vi "ElevatorStateControl.vi"(9 "Elevator State":string) -> (1 "Elevator State Out":string, 2 "Target Elevator Position":dbl, 4 "Target Vacuum Pump Power":dbl)   [LabVIEW 2018]
uses:
  Inputs_DriverStation.vi
  SensorReadings.vi
  RobotStates.vi
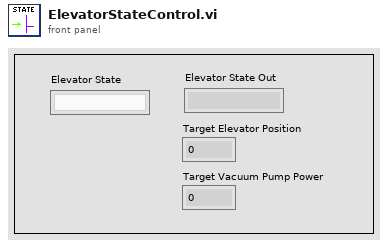
[diagram p1: front panel]
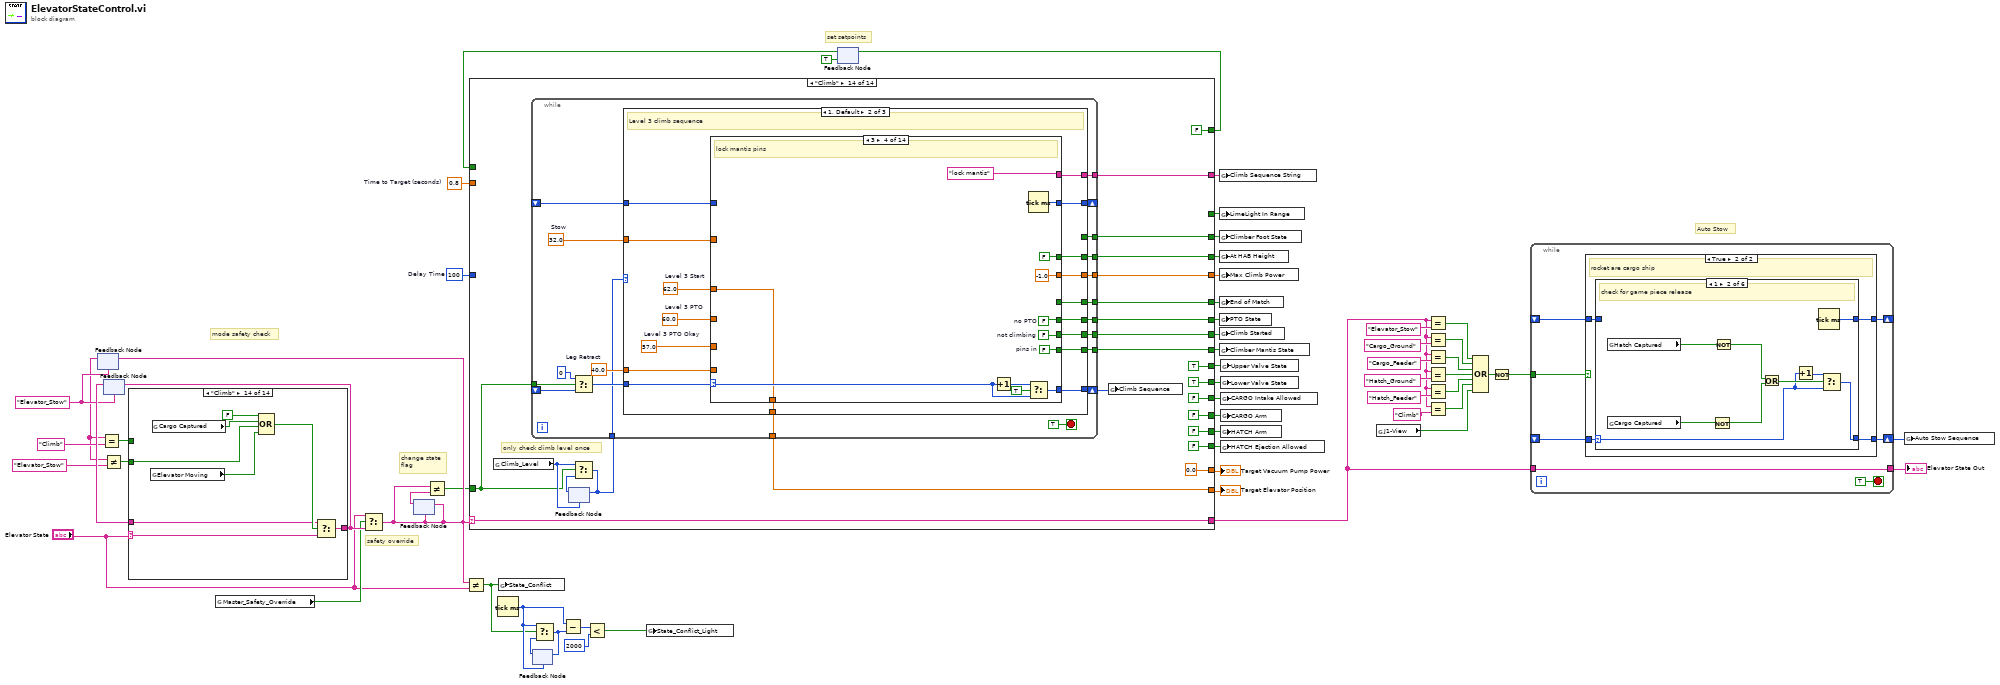
[diagram p0: block diagram]
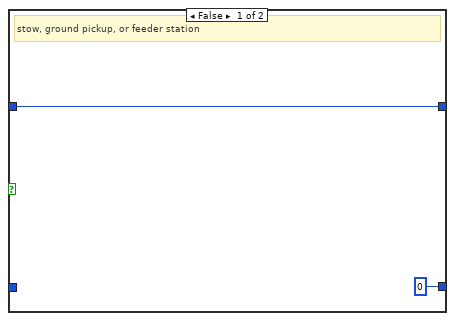
[diagram p2: hidden frame]
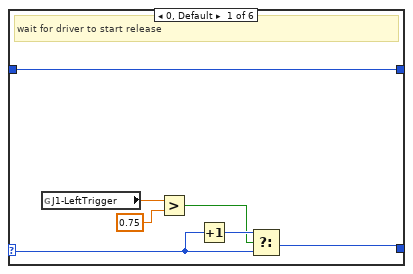
[diagram p3: hidden frame]
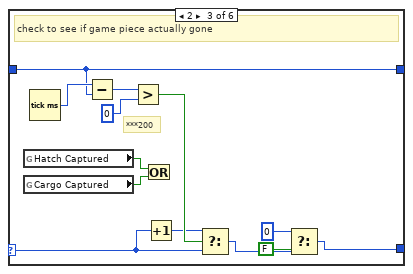
[diagram p4: hidden frame]
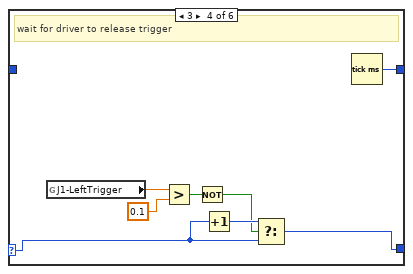
[diagram p5: hidden frame]
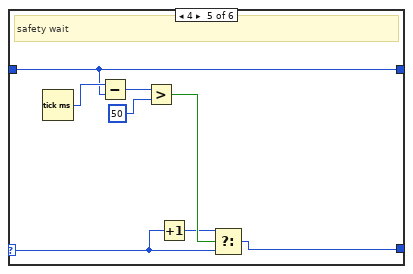
[diagram p6: hidden frame]
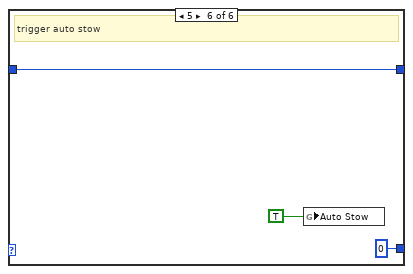
[diagram p7: hidden frame]
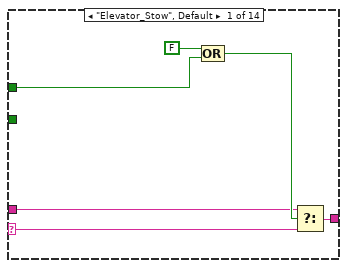
[diagram p8: hidden frame]
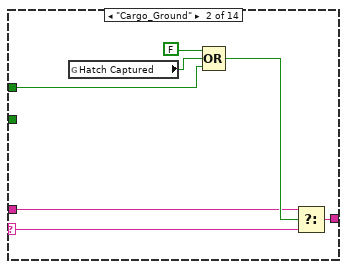
[diagram p9: hidden frame]
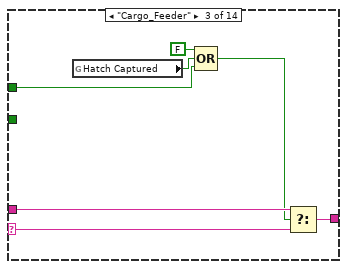
[diagram p10: hidden frame]
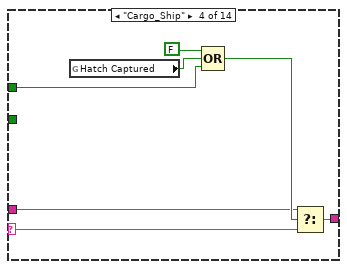
[diagram p11: hidden frame]
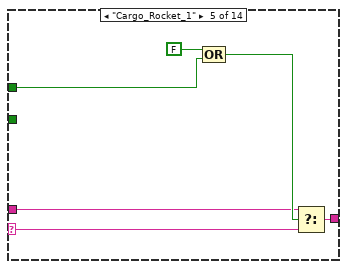
[diagram p12: hidden frame]
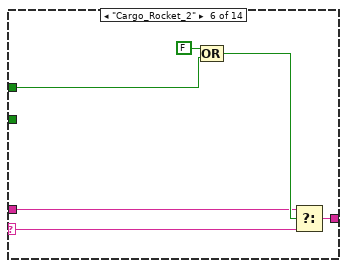
[diagram p13: hidden frame]
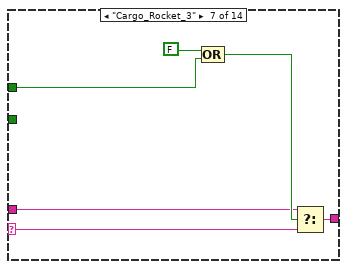
[diagram p14: hidden frame]
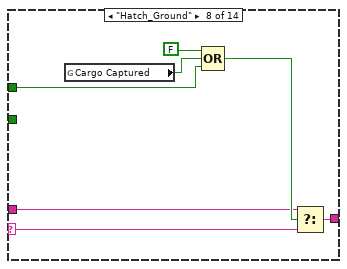
[diagram p15: hidden frame]
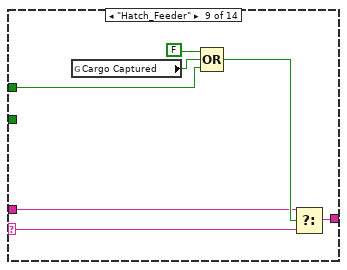
[diagram p16: hidden frame]
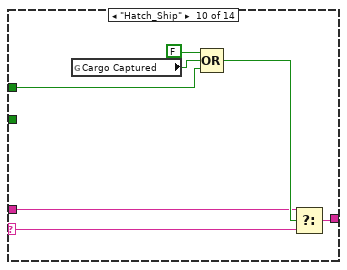
[diagram p17: hidden frame]
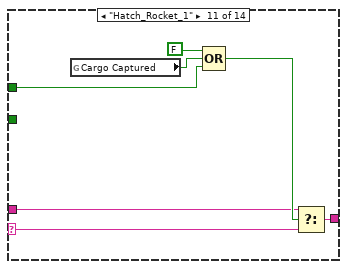
[diagram p18: hidden frame]
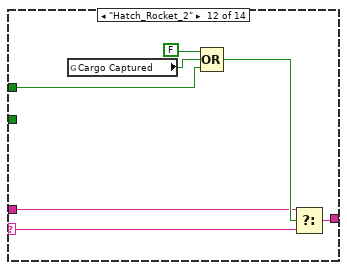
[diagram p19: hidden frame]
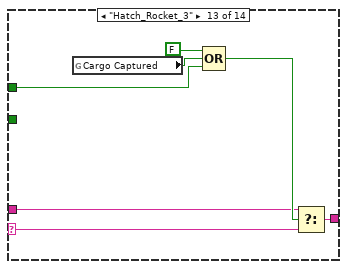
[diagram p20: hidden frame]
diagram:
  w3 = u32 100  # Delay Time
  w4 = 0.8  # Time to Target (seconds)
  w46 = "Elevator_Stow" ("Elevator State")
  # "change state\nflag"
  # "Auto Stow"
  # "safety override"
  # "mode safety check"
  # "set setpoints"
  n1 = feedback #1(w46) -> (w11:string)
  n2 = Equal?(x=w11, y="Climb") -> (x = y?=w47:bool)
  n3 = feedback #2(w46) -> (w49:string)
  n4 = Not Equal?(x=w11, y="Elevator_Stow") -> (x != y?=w10:bool)
  n5 = case shown="\"Climb\"" "Elevator State" {
    selector: "Elevator State" -> [w62 w69 w80 w83 w89 w95 w102 w108 w115 w122 w129 w136 w144 w151]
    tunnel: [w64 w71 w79 w85 w91 w97 w103 w110 w117 w124 w131 w138 w145 w152] -> w54
    tunnel: w49 -> [w63 w70 w78 w84 w90 w96 w101 w109 w116 w123 w130 w137 w143 w150]
    tunnel: w47 -> [w61 w67 w74 w81 w88 w94 w100 w106 w113 w120 w127 w134 w141 _]
    tunnel: w10 -> [_ _ _ _ _ _ _ _ _ _ _ _ _ w149]
    frame "Elevator_Stow", Default {
      n6 = Compound Arithmetic op=OR(FALSE, w61) -> (w65:bool)
      n7 = Select(t=w63, s=w65, f=w62) -> (s? t:f=w64:string)
    }
    frame "Cargo_Ground" {
      n8 = global read "SensorReadings.vi" "Hatch Captured"() -> (w68:bool)
      n9 = Compound Arithmetic op=OR(FALSE, w68, w67) -> (w72:bool)
      n10 = Select(t=w70, s=w72, f=w69) -> (s? t:f=w71:string)
    }
    frame "Cargo_Feeder" {
      n11 = global read "SensorReadings.vi" "Hatch Captured"() -> (w75:bool)
      n12 = Compound Arithmetic op=OR(FALSE, w75, w74) -> (w76:bool)
      n13 = Select(t=w78, s=w76, f=w80) -> (s? t:f=w79:string)
    }
    frame "Cargo_Ship" {
      n14 = global read "SensorReadings.vi" "Hatch Captured"() -> (w82:bool)
      n15 = Compound Arithmetic op=OR(FALSE, w82, w81) -> (w86:bool)
      n16 = Select(t=w84, s=w86, f=w83) -> (s? t:f=w85:string)
    }
    frame "Cargo_Rocket_1" {
      n17 = Compound Arithmetic op=OR(FALSE, w88) -> (w92:bool)
      n18 = Select(t=w90, s=w92, f=w89) -> (s? t:f=w91:string)
    }
    frame "Cargo_Rocket_2" {
      n19 = Compound Arithmetic op=OR(FALSE, w94) -> (w98:bool)
      n20 = Select(t=w96, s=w98, f=w95) -> (s? t:f=w97:string)
    }
    frame "Cargo_Rocket_3" {
      n21 = Compound Arithmetic op=OR(FALSE, w100) -> (w104:bool)
      n22 = Select(t=w101, s=w104, f=w102) -> (s? t:f=w103:string)
    }
    frame "Hatch_Ground" {
      n23 = global read "SensorReadings.vi" "Cargo Captured"() -> (w107:bool)
      n24 = Compound Arithmetic op=OR(FALSE, w107, w106) -> (w111:bool)
      n25 = Select(t=w109, s=w111, f=w108) -> (s? t:f=w110:string)
    }
    frame "Hatch_Feeder" {
      n26 = global read "SensorReadings.vi" "Cargo Captured"() -> (w114:bool)
      n27 = Compound Arithmetic op=OR(FALSE, w114, w113) -> (w118:bool)
      n28 = Select(t=w116, s=w118, f=w115) -> (s? t:f=w117:string)
    }
    frame "Hatch_Ship" {
      n29 = global read "SensorReadings.vi" "Cargo Captured"() -> (w121:bool)
      n30 = Compound Arithmetic op=OR(FALSE, w121, w120) -> (w125:bool)
      n31 = Select(t=w123, s=w125, f=w122) -> (s? t:f=w124:string)
    }
    frame "Hatch_Rocket_1" {
      n32 = global read "SensorReadings.vi" "Cargo Captured"() -> (w128:bool)
      n33 = Compound Arithmetic op=OR(FALSE, w128, w127) -> (w132:bool)
      n34 = Select(t=w130, s=w132, f=w129) -> (s? t:f=w131:string)
    }
    frame "Hatch_Rocket_2" {
      n35 = global read "SensorReadings.vi" "Cargo Captured"() -> (w135:bool)
      n36 = Compound Arithmetic op=OR(FALSE, w135, w134) -> (w139:bool)
      n37 = Select(t=w137, s=w139, f=w136) -> (s? t:f=w138:string)
    }
    frame "Hatch_Rocket_3" {
      n38 = global read "SensorReadings.vi" "Cargo Captured"() -> (w142:bool)
      n39 = Compound Arithmetic op=OR(FALSE, w142, w141) -> (w146:bool)
      n40 = Select(t=w143, s=w146, f=w144) -> (s? t:f=w145:string)
    }
    frame "Climb" {
      n41 = global read "RobotStates.vi" "Elevator Moving"() -> (w148:bool)
      n42 = global read "SensorReadings.vi" "Cargo Captured"() -> (w153:bool)
      n43 = Compound Arithmetic op=OR(FALSE, w153, w149, w148) -> (w154:bool)
      n44 = Select(t=w150, s=w154, f=w151) -> (s? t:f=w152:string)
    }
  }
  n45 = feedback-in #2(w54) -> ()
  n46 = global read "Inputs_DriverStation.vi" "Master_Safety_Override"() -> (w53:bool)
  n47 = Select(t="Elevator State", s=w53, f=w54) -> (s? t:f=w16:string)
  n48 = feedback-in #1(w16) -> ()
  n49 = feedback-in #3(w16) -> ()
  n50 = feedback #3(w16) -> (w17:string)
  n51 = Not Equal?(x=w16, y=w17) -> (x != y?=w15:bool)
  n52 = Not Equal?(x=w16, y="Elevator State") -> (x != y?=w22:bool)
  n53 = Tick Count (ms)() -> (millisecond timer value=w26:u32)
  n54 = global write "RobotStates.vi" "State_Conflict"(w22) -> ()
  n55 = feedback #4(w26) -> (w27:u32)
  n56 = Select(t=w26, s=w22, f=w27) -> (s? t:f=w25:u32)
  n57 = feedback-in #4(w25) -> ()
  n58 = Subtract(x=w26, y=w25) -> (x-y=w24:u32)
  n59 = Less?(x=w24, y=u32 2000) -> (x < y?=w21:bool)
  n60 = global write "RobotStates.vi" "State_Conflict_Light"(w21) -> ()
  n61 = feedback #5(TRUE) -> (w19:bool)
  n62 = case shown="\"Climb\"" w16 {
    selector: w16 -> [w179 w194 w234 w248 w289 w311 w333 w347 w409 w450 w491 w506 w521 w546]
    tunnel: [FALSE TRUE TRUE TRUE TRUE TRUE TRUE FALSE FALSE FALSE FALSE FALSE FALSE FALSE] -> w60
    tunnel: [w179 w194 w234 w248 w289 w311 w333 w347 w409 w450 w491 w506 w521 w546] -> w29
    tunnel: [w157 FALSE w197 TRUE TRUE w292 w315 FALSE FALSE FALSE FALSE FALSE FALSE FALSE] -> w59
    tunnel: [w178 32.0 w204 46.0 w275 w296 w313 32.0 w374 w436 w477 61.5 91.0 w532] -> w58
    tunnel: [FALSE FALSE FALSE FALSE FALSE FALSE FALSE TRUE w378 TRUE TRUE TRUE TRUE FALSE] -> w57
    tunnel: [w170 0.0 0.0 0.0 0.0 0.0 0.0 w343 w407 w448 w489 w502 w517 0.0 ("Vacuum_Pump")] -> w55
    tunnel: [FALSE FALSE FALSE FALSE FALSE FALSE FALSE TRUE TRUE TRUE TRUE TRUE TRUE FALSE] -> w56
    tunnel: [TRUE TRUE TRUE TRUE TRUE TRUE TRUE TRUE FALSE FALSE FALSE FALSE FALSE TRUE] -> w52
    tunnel: [TRUE TRUE TRUE TRUE TRUE TRUE TRUE FALSE TRUE TRUE TRUE TRUE TRUE TRUE] -> w51
    tunnel: [FALSE FALSE FALSE FALSE FALSE FALSE FALSE FALSE FALSE FALSE FALSE FALSE FALSE w535] -> w1
    tunnel: [w168 FALSE FALSE FALSE FALSE FALSE FALSE FALSE FALSE FALSE FALSE FALSE FALSE FALSE] -> w20
    tunnel: w19 -> [w164 _ _ _ _ _ _ _ _ _ _ _ _ _]
    tunnel: w15 -> [_ _ w212 _ _ _ _ _ w380 _ _ _ _ w534]
    tunnel: [w167 w184 w203 w238 w280 w303 w325 w338 w386 w443 w484 w497 w512 w531] -> w14
    tunnel: [w166 w183 w202 w237 w279 w302 w324 w337 w385 w442 w483 w496 w511 w530] -> w13
    tunnel: [FALSE FALSE FALSE FALSE FALSE FALSE FALSE FALSE FALSE FALSE FALSE FALSE FALSE w529] -> w9
    tunnel: [_ _ _ _ _ _ _ _ _ _ _ _ _ w527] -> w8
    tunnel: [-1.0 ("y") -1.0 ("y") -1.0 ("y") -1.0 ("y") -1.0 ("y") -1.0 ("y") -1.0 ("y") -1.0 ("y") -1.0 ("y") -1.0 ("y") -1.0 ("y") -1.0 ("y") -1.0 ("y") w526] -> w7
    tunnel: [_ _ _ _ _ _ _ _ _ _ _ _ _ w525] -> w6
    tunnel: [_ _ _ _ w267 _ _ _ w367 w429 w470 _ _ _] -> w5
    tunnel: w4 -> [_ _ _ _ w265 _ _ _ w365 w428 w468 _ _ _]
    tunnel: w3 -> [_ _ _ _ w266 _ _ _ w366 w427 w469 _ _ _]
    tunnel: [_ _ _ _ _ _ _ _ _ _ _ _ _ w524] -> w2
    frame "Elevator_Stow", Default {
      w166 = FALSE  # no PTO
      w167 = FALSE  # not climbing
      w178 = 32.0  # below 34.5 to ensure reset
      n63 = global read "Inputs_DriverStation.vi" "Reinit_Stow_Vacuum"() -> (w161:bool)
      n64 = global read "Inputs_DriverStation.vi" "Vacuum_Pump"() -> (w172:dbl)
      n65 = global read "RobotStates.vi" "Autopilot"() -> (w160:bool)
      n66 = Select(t=TRUE, s=w161, f=w164) -> (s? t:f=w163:bool)
      n67 = Select(t=w172, s=w163, f=0.0) -> (s? t:f=w170:dbl)
      n68 = Select(t=TRUE, s=w163, f=w163) -> (s? t:f=w168:bool)
      n69 = Select(t=TRUE, s=w160, f=FALSE) -> (s? t:f=w157:bool)
    }
    frame "Cargo_Ground" {
      w183 = FALSE  # no PTO
      w184 = FALSE  # not climbing
    }
    frame "Cargo_Feeder" {
      w199 = TRUE  # hold CARGO arm up
      w202 = FALSE  # no PTO
      w203 = FALSE  # not climbing
      w205 = 32.0  # gotten CARGO
      w209 = FALSE  # gotten CARGO
      w221 = -2.0  # (ft/s)
      w208 = 52.0  # getting CARGO
      w210 = TRUE  # getting CARGO
      # "autopilot"
      # "auto protect CARGO"
      n70 = global read "SensorReadings.vi" "EncoderVel_RightDrive"() -> (w225:dbl)
      n71 = global read "SensorReadings.vi" "EncoderVel_LeftDrive"() -> (w226:dbl)
      n72 = global read "SensorReadings.vi" "Cargo Captured"() -> (w219:bool)
      n73 = Add(x=w226, y=w225) -> (x+y=w224:dbl)
      n74 = Divide(x=w224, y=2.0) -> (x/y=w222:dbl)
      n75 = Less?(x=w222, y=w221) -> (x < y?=w220:bool)
      n76 = And(x=w220, y=w219) -> (x .and. y?=w218:bool)
      n77 = feedback #6(FALSE) -> (w216:bool)
      n78 = Select(t=TRUE, s=w218, f=w216) -> (s? t:f=w214:bool)
      n79 = Select(t=FALSE, s=w212, f=w214) -> (s? t:f=w207:bool)
      n80 = feedback-in #6(w207) -> ()
      n81 = Not(x=w207) -> (.not. x?=w206:bool)
      n82 = global read "RobotStates.vi" "Autopilot"() -> (w200:bool)
      n83 = Select(t=w210, s=w206, f=w209) -> (s? t:f=w198:bool)
      n84 = Select(t=w199, s=w200, f=w198) -> (s? t:f=w197:bool)
      n85 = Select(t=w208, s=w206, f=w205) -> (s? t:f=w204:dbl)
    }
    frame "Cargo_Ship" {
      w237 = FALSE  # no PTO
      w238 = FALSE  # not climbing
    }
    frame "Cargo_Rocket_1" {
      w256 = 1.5  # feet per second
      w279 = FALSE  # no PTO
      w280 = FALSE  # not climbing
      n86 = global read "SensorReadings.vi" "LimeLight Distance (in)"() -> (w254:dbl)
      n87 = global read "SensorReadings.vi" "EncoderVel_RightDrive"() -> (w263:dbl)
      n88 = global read "SensorReadings.vi" "EncoderVel_LeftDrive"() -> (w264:dbl)
      n89 = Add(x=w264, y=w263) -> (x+y=w262:dbl)
      n90 = Divide(x=w254, y=12.0) -> (x/y=w252:dbl)
      n91 = Divide(x=w262, y=2.0) -> (x/y=w257:dbl)
      n92 = In Range and Coerce(upper limit=10.0, x=w257, lower limit=w256) -> (coerced(x)=w255:dbl)  [unwired: 1 out]
      n93 = Divide(x=w252, y=w255) -> (x/y=w259:dbl)
      n94 = Greater Than 0?(x=w259) -> (x > 0?=w260:bool)
      n95 = Select(t=w259, s=w260, f=inf) -> (s? t:f=w251:dbl)
      n96 = global read "SensorReadings.vi" "LimeLight Valid"() -> (w270:bool)
      n97 = Select(t=w251, s=w270, f=inf) -> (s? t:f=w269:dbl)
      n98 = call "TimeBelowThreshold.vi"("Current Value"=w269, "Threshold"=w265) -> ("Time Below"=w271:u32)  [unwired: 3 in]
      n99 = global read "RobotStates.vi" "Autopilot"() -> (w277:bool)
      n100 = Greater?(x=w271, y=w266) -> (0:w272:bool)
      n101 = call "RisingEdgeTrigger.vi"("Raw Signal"=w272) -> ("Trigger"=w267:bool)
      n102 = Select(t=45.0, s=w277, f=32.0) -> (s? t:f=w275:dbl)
    }
    frame "Cargo_Rocket_2" {
      w302 = FALSE  # no PTO
      w303 = FALSE  # not climbing
      w296 = 62.5
      n103 = global read "SensorReadings.vi" "EncoderPos_Elevator"() -> (w297:dbl)
      n104 = Subtract(x=w297, y=w296) -> (x-y=w295:dbl)
      n105 = Absolute Value(x=w295) -> (abs(x)=w291:dbl)
      n106 = Less?(x=w291, y=10.0) -> (x < y?=w293:bool)
      n107 = Select(t=TRUE, s=w293, f=FALSE) -> (s? t:f=w292:bool)
    }
    frame "Cargo_Rocket_3" {
      w324 = FALSE  # no PTO
      w325 = FALSE  # not climbing
      w313 = 91.0
      n108 = global read "SensorReadings.vi" "EncoderPos_Elevator"() -> (w319:dbl)
      n109 = Subtract(x=w319, y=w313) -> (x-y=w318:dbl)
      n110 = Absolute Value(x=w318) -> (abs(x)=w316:dbl)
      n111 = Less?(x=w316, y=10.0) -> (x < y?=w317:bool)
      n112 = Select(t=TRUE, s=w317, f=FALSE) -> (s? t:f=w315:bool)
    }
    frame "Hatch_Ground" {
      w337 = FALSE  # no PTO
      w338 = FALSE  # not climbing
      n113 = global read "Inputs_DriverStation.vi" "Vacuum_Pump"() -> (w343:dbl)
    }
    frame "Hatch_Feeder" {
      w355 = 2.0  # feet per second
      w385 = FALSE  # no PTO
      w386 = FALSE  # not climbing
      w396 = -2.0  # (ft/s)
      w388 = FALSE  # gotten HATCH
      w402 = TRUE  # to get HATCH
      # "auto protect HATCH"
      n114 = global read "SensorReadings.vi" "EncoderVel_RightDrive"() -> (w400:dbl)
      n115 = global read "SensorReadings.vi" "EncoderVel_LeftDrive"() -> (w401:dbl)
      n116 = global read "SensorReadings.vi" "LimeLight Distance (in)"() -> (w353:dbl)
      n117 = global read "SensorReadings.vi" "EncoderVel_RightDrive"() -> (w363:dbl)
      n118 = global read "SensorReadings.vi" "EncoderVel_LeftDrive"() -> (w364:dbl)
      n119 = global read "SensorReadings.vi" "Hatch Captured"() -> (w382:bool)
      n120 = Add(x=w401, y=w400) -> (x+y=w399:dbl)
      n121 = Divide(x=w399, y=2.0) -> (x/y=w397:dbl)
      n122 = Less?(x=w397, y=w396) -> (x < y?=w395:bool)
      n123 = Add(x=w364, y=w363) -> (x+y=w362:dbl)
      n124 = And(x=w395, y=w382) -> (x .and. y?=w394:bool)
      n125 = Not(x=w382) -> (.not. x?=w381:bool)
      n126 = Divide(x=w353, y=12.0) -> (x/y=w351:dbl)
      n127 = Divide(x=w362, y=2.0) -> (x/y=w356:dbl)
      n128 = Or(x=w381, y=w380) -> (x .or. y?=w379:bool)
      n129 = feedback #7(FALSE) -> (w392:bool)
      n130 = Select(t=TRUE, s=w394, f=w392) -> (s? t:f=w390:bool)
      n131 = In Range and Coerce(upper limit=10.0 ("feet per second"), x=w356, lower limit=w355) -> (coerced(x)=w354:dbl)  [unwired: 1 out]
      n132 = Select(t=FALSE, s=w379, f=w390) -> (s? t:f=w387:bool)
      n133 = feedback-in #7(w387) -> ()
      n134 = Divide(x=w351, y=w354) -> (x/y=w359:dbl)
      n135 = Not(x=w387) -> (.not. x?=w383:bool)
      n136 = Greater Than 0?(x=w359) -> (x > 0?=w360:bool)
      n137 = Select(t=w359, s=w360, f=inf) -> (s? t:f=w357:dbl)
      n138 = global read "SensorReadings.vi" "LimeLight Valid"() -> (w371:bool)
      n139 = Select(t=w402, s=w383, f=w388) -> (s? t:f=w378:bool)
      n140 = Select(t=w357, s=w371, f=inf) -> (s? t:f=w372:dbl)
      n141 = global read "RobotStates.vi" "Autopilot"() -> (w377:bool)
      n142 = call "TimeBelowThreshold.vi"("Current Value"=w372, "Threshold"=w365) -> ("Time Below"=w369:u32)  [unwired: 3 in]
      n143 = global read "Inputs_DriverStation.vi" "Vacuum_Pump"() -> (w407:dbl)
      n144 = Greater?(x=w369, y=w366) -> (0:w368:bool)
      n145 = Select(t=55.0, s=w377, f=32.0) -> (s? t:f=w374:dbl)
      n146 = call "RisingEdgeTrigger.vi"("Raw Signal"=w368) -> ("Trigger"=w367:bool)
    }
    frame "Hatch_Ship" {
      w418 = 2.0  # feet per second
      w442 = FALSE  # no PTO
      w443 = FALSE  # not climbing
      n147 = global read "SensorReadings.vi" "LimeLight Distance (in)"() -> (w416:dbl)
      n148 = global read "SensorReadings.vi" "EncoderVel_RightDrive"() -> (w425:dbl)
      n149 = global read "SensorReadings.vi" "EncoderVel_LeftDrive"() -> (w426:dbl)
      n150 = Add(x=w426, y=w425) -> (x+y=w424:dbl)
      n151 = Divide(x=w416, y=12.0) -> (x/y=w414:dbl)
      n152 = Divide(x=w424, y=2.0) -> (x/y=w419:dbl)
      n153 = In Range and Coerce(upper limit=10.0, x=w419, lower limit=w418) -> (coerced(x)=w417:dbl)  [unwired: 1 out]
      n154 = Divide(x=w414, y=w417) -> (x/y=w421:dbl)
      n155 = Greater Than 0?(x=w421) -> (x > 0?=w422:bool)
      n156 = Select(t=w421, s=w422, f=inf) -> (s? t:f=w413:dbl)
      n157 = global read "SensorReadings.vi" "LimeLight Valid"() -> (w433:bool)
      n158 = Select(t=w413, s=w433, f=inf) -> (s? t:f=w434:dbl)
      n159 = call "TimeBelowThreshold.vi"("Current Value"=w434, "Threshold"=w428) -> ("Time Below"=w431:u32)  [unwired: 3 in]
      n160 = global read "RobotStates.vi" "Autopilot"() -> (w439:bool)
      n161 = global read "Inputs_DriverStation.vi" "Vacuum_Pump"() -> (w448:dbl)
      n162 = Greater?(x=w431, y=w427) -> (0:w430:bool)
      n163 = call "RisingEdgeTrigger.vi"("Raw Signal"=w430) -> ("Trigger"=w429:bool)
      n164 = Select(t=55.0, s=w439, f=32.0) -> (s? t:f=w436:dbl)
    }
    frame "Hatch_Rocket_1" {
      w459 = 2.0  # feet per second
      w483 = FALSE  # no PTO
      w484 = FALSE  # not climbing
      # "autopilot"
      n165 = global read "SensorReadings.vi" "LimeLight Distance (in)"() -> (w457:dbl)
      n166 = global read "SensorReadings.vi" "EncoderVel_RightDrive"() -> (w466:dbl)
      n167 = global read "SensorReadings.vi" "EncoderVel_LeftDrive"() -> (w467:dbl)
      n168 = Add(x=w467, y=w466) -> (x+y=w465:dbl)
      n169 = Divide(x=w457, y=12.0) -> (x/y=w455:dbl)
      n170 = Divide(x=w465, y=2.0) -> (x/y=w460:dbl)
      n171 = In Range and Coerce(upper limit=10.0, x=w460, lower limit=w459) -> (coerced(x)=w458:dbl)  [unwired: 1 out]
      n172 = Divide(x=w455, y=w458) -> (x/y=w462:dbl)
      n173 = Greater Than 0?(x=w462) -> (x > 0?=w463:bool)
      n174 = Select(t=w462, s=w463, f=inf) -> (s? t:f=w454:dbl)
      n175 = global read "SensorReadings.vi" "LimeLight Valid"() -> (w473:bool)
      n176 = Select(t=w454, s=w473, f=inf) -> (s? t:f=w472:dbl)
      n177 = call "TimeBelowThreshold.vi"("Current Value"=w472, "Threshold"=w468) -> ("Time Below"=w474:u32)  [unwired: 3 in]
      n178 = Greater?(x=w474, y=w469) -> (0:w475:bool)
      n179 = global read "RobotStates.vi" "Autopilot"() -> (w480:bool)
      n180 = global read "Inputs_DriverStation.vi" "Vacuum_Pump"() -> (w489:dbl)
      n181 = call "RisingEdgeTrigger.vi"("Raw Signal"=w475) -> ("Trigger"=w470:bool)
      n182 = Select(t=55.0, s=w480, f=32.0) -> (s? t:f=w477:dbl)
    }
    frame "Hatch_Rocket_2" {
      w496 = FALSE  # no PTO
      w497 = FALSE  # not climbing
      n183 = global read "Inputs_DriverStation.vi" "Vacuum_Pump"() -> (w502:dbl)
    }
    frame "Hatch_Rocket_3" {
      w511 = FALSE  # no PTO
      w512 = FALSE  # not climbing
      n184 = global read "Inputs_DriverStation.vi" "Vacuum_Pump"() -> (w517:dbl)
    }
    frame "Climb" {
      # "only check climb level once"
      n185 = global read "Inputs_DriverStation.vi" "Climb_Level"() -> (w536:u8)
      n186 = feedback #8(w536) -> (w537:u8)
      n187 = Select(t=w536, s=w534, f=w537) -> (s? t:f=w533:u8)
      n188 = while {
        shift-right: [w565] -> w528
        shift-left: _ -> [w561]
        shift-right: [w564] -> _
        shift-left: _ -> [w563]
        tunnel: [w562] -> w535
        tunnel: w534 -> [w559]
        tunnel: w533 -> [w552]
        tunnel: [w554] -> w532
        tunnel: [w557] -> w531
        tunnel: [w556] -> w530
        tunnel: [w555] -> w529
        tunnel: [w551] -> w527
        tunnel: [w550] -> w526
        tunnel: [w549] -> w525
        tunnel: [w547] -> w524
        stop <- TRUE stop-if-true
        w548 = 32.0  # Stow
        w553 = 40.0  # Leg Retract
        n189 = Select(t=0, s=w559, f=w561) -> (s? t:f=w560:i32)
        n190 = case shown="1, Default" w552 {
          tunnel: [w578 w831 w1054] -> w565
          tunnel: [w582 w838 w1061] -> w564
          tunnel: w563 -> [w584 w839 w1062]
          tunnel: [w577 w832 w1055] -> w562
          tunnel: w560 -> [w580 w837 w1060]
          tunnel: [w575 w833 w1056] -> w557
          tunnel: [w576 w834 w1057] -> w556
          tunnel: [w579 w835 w1058] -> w555
          tunnel: [w574 w830 w1053] -> w554
          tunnel: w553 -> [w581 w836 w1059]
          tunnel: [w583 w829 w1052] -> w551
          tunnel: [w573 w827 w1050] -> w550
          tunnel: [w572 w825 w1048] -> w549
          tunnel: w548 -> [w567 w824 w1047]
          tunnel: [_ _ w1046] -> w547
          frame 0 {
            w571 = 45.0  # Level 2 Pre-Climb
            w568 = 39.5  # Level 2 PTO Okay
            w570 = 45.5  # Level 2 Start
            w569 = 42.5  # Level 2 PTO
            # "Level 2 climb sequence"
            n191 = case shown="1" w580 {
              selector: w580 -> [w594 w609 w624 w641 w652 w673 w684 w703 w722 w733 w751 w760 w775 w787 w804 w818]
              tunnel: [w596 w611 w619 w640 w651 w672 w686 w705 w721 w732 w750 w759 w774 w786 w803 w818] -> w578
              tunnel: [w593 w599 w617 w638 w654 w665 w685 w704 w717 w725 w738 w763 w777 w789 w811 w821] -> w582
              tunnel: w584 -> [_ w599 w617 _ w654 w665 w685 w704 w717 _ w738 w763 w777 w789 w811 w821]
              tunnel: [w592 w608 w630 w639 w650 w675 w689 w708 w724 w735 w753 w764 w778 w790 w812 w822] -> w577
              tunnel: [w585 w597 w612 w631 w643 w658 _ w693 _ _ _ _ w770 w785 w806 w815] -> w574
              tunnel: [w590 w607 w618 w636 w649 w668 w690 w709 w720 w731 w749 w765 w779 w791 w813 w823] -> w575
              tunnel: [w589 w606 w616 w635 w648 w667 w691 w710 w719 w730 w748 w758 w773 w783 w809 w819] -> w576
              tunnel: [FALSE FALSE FALSE FALSE FALSE FALSE FALSE FALSE FALSE FALSE FALSE w762 TRUE TRUE TRUE FALSE] -> w579
              tunnel: w581 -> [_ _ _ _ _ _ _ _ _ _ _ _ w770 w785 w806 w815]
              tunnel: ["release mantis" "wait for mantis to deploy" "wait for elevator to reach climb height" "lock mantis" "confirm mantis lock" "wait for the driver to start climbing #1" "wait for driver to raise elevator" "wait for elevator to reach start height" "wait for elevator to pass PTO height" "engage the PTO" "ensure PTO is engaged" "wait for the robot to be on HAB" "stop climbing" "wait to disengage PTO" "retract the legs after confirm " "elevator powered down"] -> w583
              tunnel: [-1.0 ("y") -1.0 ("y") -1.0 ("y") -1.0 ("y") -1.0 ("y") -1.0 ("y") -1.0 ("y") -1.0 ("y") -0.05 ("y") -0.05 ("y") -0.05 ("y") -1.0 ("y") -1.0 ("y") -1.0 ("y") -1.0 ("y") -1.0 ("y")] -> w573
              tunnel: [_ _ _ _ _ _ _ _ _ _ _ _ _ _ _ w814] -> w572
              tunnel: w571 -> [_ _ w612 w631 w643 w658 _ _ _ _ _ _ _ _ _ _]
              tunnel: w570 -> [_ _ _ _ _ _ _ w693 _ _ _ _ _ _ _ _]
              tunnel: w569 -> [_ _ _ _ _ _ _ _ w712 _ _ _ _ _ _ _]
              tunnel: w568 -> [_ _ _ _ _ _ _ _ _ _ w736 _ _ _ _ _]
              tunnel: w567 -> [w585 w597 _ _ _ _ _ _ _ _ _ _ _ _ _ _]
              frame 0, Default {
                w589 = FALSE  # no PTO
                w590 = FALSE  # not climbing
                w592 = TRUE  # pins out
                # "release mantis pins and command to climb height"
                n192 = Increment(x=w594) -> (x+1=w595:i32)
                n193 = Select(t=w595, s=TRUE, f=w594) -> (s? t:f=w596:i32)
                n194 = Tick Count (ms)() -> (millisecond timer value=w593:u32)
              }
              frame 1 {
                w606 = FALSE  # no PTO
                w607 = FALSE  # not climbing
                w608 = TRUE  # pins out
                # "wait for mantis to deploy"
                n195 = Tick Count (ms)() -> (millisecond timer value=w602:u32)
                n196 = Subtract(x=w602, y=w599) -> (x-y=w601:u32)
                n197 = Greater?(x=w601, y=u32 0) -> (0:w598:bool)
                n198 = Increment(x=w609) -> (x+1=w610:i32)
                n199 = Select(t=w610, s=w598, f=w609) -> (s? t:f=w611:i32)
              }
              frame 2 {
                w616 = FALSE  # no PTO
                w618 = FALSE  # not climbing
                w630 = TRUE  # pins out
                # "wait for elevator to start moving\nand then stop moving"
                # "wait for elevator to reach climb position"
                n200 = global read "RobotStates.vi" "Elevator Moving"() -> (w622:bool)
                n201 = call "RisingEdgeTrigger.vi"("Raw Signal"=w622) -> ("Trigger"=w629:bool)
                n202 = Not(x=w622) -> (.not. x?=w621:bool)
                n203 = feedback #9(FALSE) -> (w627:bool)
                n204 = Select(t=TRUE, s=w629, f=w627) -> (s? t:f=w623:bool)
                n205 = feedback-in #9(w623) -> ()
                n206 = And(x=w623, y=w621) -> (x .and. y?=w620:bool)
                n207 = Increment(x=w624) -> (x+1=w625:i32)
                n208 = Select(t=w625, s=w620, f=w624) -> (s? t:f=w619:i32)
              }
              frame 3 {
                w635 = FALSE  # no PTO
                w636 = FALSE  # not climbing
                w639 = FALSE  # pins in
                # "lock mantis pins"
                n209 = Increment(x=w641) -> (x+1=w642:i32)
                n210 = Tick Count (ms)() -> (millisecond timer value=w638:u32)
                n211 = Select(t=w642, s=TRUE, f=w641) -> (s? t:f=w640:i32)
              }
              frame 4 {
                w648 = FALSE  # no PTO
                w649 = FALSE  # not climbing
                w650 = FALSE  # pins in
                # "wait for mantis legs to lock"
                n212 = Tick Count (ms)() -> (millisecond timer value=w657:u32)
                n213 = Subtract(x=w657, y=w654) -> (x-y=w656:u32)
                n214 = Greater?(x=w656, y=u32 500) -> (0:w646:bool)
                n215 = Increment(x=w652) -> (x+1=w653:i32)
                n216 = Select(t=w653, s=w646, f=w652) -> (s? t:f=w651:i32)
              }
              frame 5 {
                w667 = FALSE  # no PTO
                w668 = FALSE  # not climbing
                w675 = FALSE  # pins in
                # "wait for the driver to start climbing"
                n217 = global read "Inputs_DriverStation.vi" "J1-RightTrigger"() -> (w664:dbl)
                n218 = Greater?(x=w664, y=0.2) -> (0:w662:bool)
                n219 = feedback #10(FALSE) -> (w669:bool)
                n220 = Select(t=TRUE, s=w662, f=w669) -> (s? t:f=w661:bool)
                n221 = feedback-in #10(w661) -> ()
                n222 = Increment(x=w673) -> (x+1=w674:i32)
                n223 = Select(t=w674, s=w661, f=w673) -> (s? t:f=w672:i32)
              }
              frame 6 {
                w691 = FALSE  # no PTO
                w690 = TRUE  # climbing
                w689 = FALSE  # pins in
                # "Lower elevator contacts HAB first time"
                n224 = global read "Inputs_DriverStation.vi" "J1-LeftTrigger"() -> (w680:dbl)
                n225 = Greater?(x=w680, y=0.75) -> (0:w678:bool)
                n226 = feedback #11(FALSE) -> (w681:bool)
                n227 = Select(t=TRUE, s=w678, f=w681) -> (s? t:f=w677:bool)
                n228 = feedback-in #11(w677) -> ()
                n229 = Increment(x=w684) -> (x+1=w687:i32)
                n230 = Select(t=w687, s=w677, f=w684) -> (s? t:f=w686:i32)
              }
              frame 7 {
                w710 = FALSE  # no PTO
                w709 = FALSE  # not climbing
                w708 = FALSE  # pins in
                # "Wait for elevator to reach start height"
                n231 = global read "RobotStates.vi" "Elevator Moving"() -> (w696:bool)
                n232 = call "RisingEdgeTrigger.vi"("Raw Signal"=w696) -> ("Trigger"=w701:bool)
                n233 = Not(x=w696) -> (.not. x?=w695:bool)
                n234 = feedback #12(FALSE) -> (w699:bool)
                n235 = Select(t=TRUE, s=w701, f=w699) -> (s? t:f=w697:bool)
                n236 = feedback-in #12(w697) -> ()
                n237 = And(x=w697, y=w695) -> (x .and. y?=w694:bool)
                n238 = Increment(x=w703) -> (x+1=w706:i32)
                n239 = Select(t=w706, s=w694, f=w703) -> (s? t:f=w705:i32)
              }
              frame 8 {
                w719 = FALSE  # no PTO
                w720 = TRUE  # climbing
                w724 = FALSE  # pins in
                # "wait for elevator to pass PTO height"
                n240 = global read "SensorReadings.vi" "EncoderPos_Elevator"() -> (w713:dbl)
                n241 = Less Or Equal?(x=w713, y=w712) -> (x <= y?=w714:bool)
                n242 = Increment(x=w722) -> (x+1=w723:i32)
                n243 = Select(t=w723, s=w714, f=w722) -> (s? t:f=w721:i32)
              }
              frame 9 {
                w730 = TRUE  # PTO
                w731 = TRUE  # climbing
                w735 = FALSE  # pins in
                # "engage the PTO"
                n244 = Increment(x=w733) -> (x+1=w734:i32)
                n245 = Tick Count (ms)() -> (millisecond timer value=w725:u32)
                n246 = Select(t=w734, s=TRUE, f=w733) -> (s? t:f=w732:i32)
              }
              frame 10 {
                w748 = TRUE  # PTO
                w749 = TRUE  # climbing
                w753 = FALSE  # pins in
                # "timeout"
                # "ensure PTO is engaged"
                n247 = global read "SensorReadings.vi" "EncoderPos_Elevator"() -> (w744:dbl)
                n248 = Tick Count (ms)() -> (millisecond timer value=w741:u32)
                n249 = Less Or Equal?(x=w744, y=w736) -> (x <= y?=w743:bool)
                n250 = Subtract(x=w741, y=w738) -> (x-y=w740:u32)
                n251 = Greater?(x=w740, y=u32 1000) -> (0:w737:bool)
                n252 = Or(x=w737, y=w743) -> (x .or. y?=w742:bool)
                n253 = Increment(x=w751) -> (x+1=w752:i32)
                n254 = Select(t=w752, s=w742, f=w751) -> (s? t:f=w750:i32)
              }
              frame 11 {
                w758 = TRUE  # PTO
                w765 = TRUE  # climbing
                w764 = FALSE  # pins in
                # "wait for robot to be secure on HAB"
                n255 = global read "Inputs_DriverStation.vi" "Master_Safety_Override"() -> (w766:bool)
                n256 = global read "SensorReadings.vi" "Robot On Ground"() -> (w754:bool)
                n257 = global read "Inputs_DriverStation.vi" "J1-Menu"() -> (w767:bool)
                n258 = Or(x=w754, y=w766) -> (x .or. y?=w762:bool)
                n259 = And(x=w767, y=w762) -> (x .and. y?=w757:bool)
                n260 = Increment(x=w760) -> (x+1=w761:i32)
                n261 = Select(t=w761, s=w757, f=w760) -> (s? t:f=w759:i32)
              }
              frame 12 {
                w773 = TRUE  # PTO
                w779 = FALSE  # not climbing
                w778 = FALSE  # pins in
                # "stop \"climbing\""
                n262 = Increment(x=w775) -> (x+1=w776:i32)
                n263 = Select(t=w776, s=TRUE, f=w775) -> (s? t:f=w774:i32)
              }
              frame 13 {
                w783 = TRUE  # PTO
                w791 = FALSE  # not climbing
                w790 = FALSE  # pins in
                # "wait to disengage PTO"
                n264 = Increment(x=w787) -> (x+1=w788:i32)
                n265 = Select(t=w788, s=TRUE, f=w787) -> (s? t:f=w786:i32)
              }
              frame 14 {
                w809 = FALSE  # no PTO
                w813 = FALSE  # not climbing
                w812 = FALSE  # pins in
                # "retract legs"
                n266 = global read "Inputs_DriverStation.vi" "J1-Menu"() -> (w793:bool)
                n267 = Not(x=w793) -> (.not. x?=w794:bool)
                n268 = feedback #13(FALSE ("PTO")) -> (w797:bool)
                n269 = Select(t=TRUE ("no PTO"), s=w794, f=w797) -> (s? t:f=w792:bool)
                n270 = feedback-in #13(w792) -> ()
                n271 = And(x=w792, y=w793) -> (x .and. y?=w795:bool)
                n272 = feedback #14(FALSE ("PTO")) -> (w801:bool)
                n273 = Select(t=TRUE ("no PTO"), s=w795, f=w801) -> (s? t:f=w799:bool)
                n274 = feedback-in #14(w799) -> ()
                n275 = Increment(x=w804) -> (x+1=w805:i32)
                n276 = Select(t=w805, s=w799, f=w804) -> (s? t:f=w803:i32)
              }
              frame 15 {
                w814 = TRUE  # end of match
                w819 = FALSE  # no PTO
                w823 = FALSE  # not climbing
                w822 = FALSE  # pins in
                # "turn off the elevator"
              }
            }
          }
          frame 1, Default {
            w826 = 57.0  # Level 3 PTO Okay
            w828 = 62.0  # Level 3 Start
            w840 = 60.0  # Level 3 PTO
            # "Level 3 climb sequence"
            n277 = case shown="3" w837 {
              selector: w837 -> [w850 w865 w880 w897 w908 w929 w942 w954 w973 w982 w997 w1009 w1026 w1040]
              tunnel: [w852 w867 w875 w896 w907 w928 w941 w953 w972 w981 w996 w1008 w1025 w1040] -> w831
              tunnel: [w849 w855 w873 w894 w910 w921 w937 w945 w958 w985 w999 w1011 w1033 w1043] -> w838
              tunnel: w839 -> [_ w855 w873 _ w910 w921 w937 _ w958 w985 w999 w1011 w1033 w1043]
              tunnel: [w848 w864 w886 w895 w906 w931 w944 w956 w975 w986 w1000 w1012 w1034 w1044] -> w832
              tunnel: [w841 w853 w869 w888 w900 w915 _ w948 w968 _ w992 w1007 w1028 w1037] -> w830
              tunnel: w840 -> [_ _ _ _ _ _ w934 w948 w968 _ _ _ _ _]
              tunnel: [w846 w863 w874 w892 w905 w924 w940 w952 w971 w987 w1001 w1013 w1035 w1045] -> w833
              tunnel: [w845 w862 w872 w891 w904 w923 w939 w951 w970 w980 w995 w1005 w1031 w1041] -> w834
              tunnel: [FALSE FALSE FALSE FALSE FALSE FALSE FALSE FALSE FALSE w984 TRUE TRUE TRUE FALSE] -> w835
              tunnel: w836 -> [_ _ _ _ _ _ _ _ _ _ w992 w1007 w1028 w1037]
              tunnel: ["release mantis" "wait for mantis to deploy" "wait for elevator to reach climb height" "lock mantis" "confirm mantis lock" "wait for the driver to start climbing" "wait for elevator to pass PTO height" "engage the PTO" "ensure PTO is engaged" "wait for the robot to be on HAB" "stop climbing" "wait to disengage PTO" "retract the legs after confirm " "elevator powered down"] -> w829
              tunnel: w828 -> [_ _ w869 w888 w900 w915 _ _ _ _ _ _ _ _]
              tunnel: [-1.0 ("y") -1.0 ("y") -1.0 ("y") -1.0 ("y") -1.0 ("y") -1.0 ("y") -0.05 ("y") -0.05 ("y") -0.05 ("y") -1.0 ("y") -1.0 ("y") -1.0 ("y") -1.0 ("y") -1.0 ("y")] -> w827
              tunnel: w826 -> [_ _ _ _ _ _ _ _ w964 _ _ _ _ _]
              tunnel: [_ _ _ _ _ _ _ _ _ _ _ _ _ w1036] -> w825
              tunnel: w824 -> [w841 w853 _ _ _ _ _ _ _ _ _ _ _ _]
              frame 0, Default {
                w845 = FALSE  # no PTO
                w846 = FALSE  # not climbing
                w848 = TRUE  # pins out
                # "release mantis pins and command to climb height"
                n278 = Increment(x=w850) -> (x+1=w851:i32)
                n279 = Select(t=w851, s=TRUE, f=w850) -> (s? t:f=w852:i32)
                n280 = Tick Count (ms)() -> (millisecond timer value=w849:u32)
              }
              frame 1 {
                w862 = FALSE  # no PTO
                w863 = FALSE  # not climbing
                w864 = TRUE  # pins out
                # "wait for mantis to deploy"
                n281 = Tick Count (ms)() -> (millisecond timer value=w858:u32)
                n282 = Subtract(x=w858, y=w855) -> (x-y=w857:u32)
                n283 = Greater?(x=w857, y=u32 250) -> (0:w854:bool)
                n284 = Increment(x=w865) -> (x+1=w866:i32)
                n285 = Select(t=w866, s=w854, f=w865) -> (s? t:f=w867:i32)
              }
              frame 2 {
                w872 = FALSE  # no PTO
                w874 = FALSE  # not climbing
                w886 = TRUE  # pins out
                # "wait for elevator to start moving\nand then stop moving"
                # "wait for elevator to reach climb position"
                n286 = global read "RobotStates.vi" "Elevator Moving"() -> (w878:bool)
                n287 = call "RisingEdgeTrigger.vi"("Raw Signal"=w878) -> ("Trigger"=w885:bool)
                n288 = Not(x=w878) -> (.not. x?=w877:bool)
                n289 = feedback #15(FALSE) -> (w883:bool)
                n290 = Select(t=TRUE, s=w885, f=w883) -> (s? t:f=w879:bool)
                n291 = feedback-in #15(w879) -> ()
                n292 = And(x=w879, y=w877) -> (x .and. y?=w876:bool)
                n293 = Increment(x=w880) -> (x+1=w881:i32)
                n294 = Select(t=w881, s=w876, f=w880) -> (s? t:f=w875:i32)
              }
              frame 3 {
                w891 = FALSE  # no PTO
                w892 = FALSE  # not climbing
                w895 = FALSE  # pins in
                # "lock mantis pins"
                n295 = Increment(x=w897) -> (x+1=w898:i32)
                n296 = Tick Count (ms)() -> (millisecond timer value=w894:u32)
                n297 = Select(t=w898, s=TRUE, f=w897) -> (s? t:f=w896:i32)
              }
              frame 4 {
                w904 = FALSE  # no PTO
                w905 = FALSE  # not climbing
                w906 = FALSE  # pins in
                # "wait for mantis legs to lock"
                n298 = Tick Count (ms)() -> (millisecond timer value=w913:u32)
                n299 = Subtract(x=w913, y=w910) -> (x-y=w912:u32)
                n300 = Greater?(x=w912, y=u32 500) -> (0:w902:bool)
                n301 = Increment(x=w908) -> (x+1=w909:i32)
                n302 = Select(t=w909, s=w902, f=w908) -> (s? t:f=w907:i32)
              }
              frame 5 {
                w923 = FALSE  # no PTO
                w924 = FALSE  # not climbing
                w931 = FALSE  # pins in
                # "wait for the driver to start climbing"
                n303 = global read "Inputs_DriverStation.vi" "J1-RightTrigger"() -> (w920:dbl)
                n304 = Greater?(x=w920, y=0.2) -> (0:w918:bool)
                n305 = feedback #16(FALSE) -> (w925:bool)
                n306 = Select(t=TRUE, s=w918, f=w925) -> (s? t:f=w917:bool)
                n307 = feedback-in #16(w917) -> ()
                n308 = Increment(x=w929) -> (x+1=w930:i32)
                n309 = Select(t=w930, s=w917, f=w929) -> (s? t:f=w928:i32)
              }
              frame 6 {
                w939 = FALSE  # no PTO
                w940 = TRUE  # climbing
                w944 = FALSE  # pins in
                # "wait for elevator to pass PTO height"
                n310 = global read "SensorReadings.vi" "EncoderPos_Elevator"() -> (w932:dbl)
                n311 = Less Or Equal?(x=w932, y=w934) -> (x <= y?=w933:bool)
                n312 = Increment(x=w942) -> (x+1=w943:i32)
                n313 = Select(t=w943, s=w933, f=w942) -> (s? t:f=w941:i32)
              }
              frame 7 {
                w951 = TRUE  # PTO
                w952 = TRUE  # climbing
                w956 = FALSE  # pins in
                # "engage the PTO"
                n314 = Increment(x=w954) -> (x+1=w955:i32)
                n315 = Tick Count (ms)() -> (millisecond timer value=w945:u32)
                n316 = Select(t=w955, s=TRUE, f=w954) -> (s? t:f=w953:i32)
              }
              frame 8 {
                w970 = TRUE  # PTO
                w971 = TRUE  # climbing
                w975 = FALSE  # pins in
                # "timeout"
                # "ensure PTO is engaged"
                n317 = global read "SensorReadings.vi" "EncoderPos_Elevator"() -> (w965:dbl)
                n318 = Tick Count (ms)() -> (millisecond timer value=w961:u32)
                n319 = Less Or Equal?(x=w965, y=w964) -> (x <= y?=w963:bool)
                n320 = Subtract(x=w961, y=w958) -> (x-y=w960:u32)
                n321 = Greater?(x=w960, y=u32 1000) -> (0:w957:bool)
                n322 = Or(x=w957, y=w963) -> (x .or. y?=w962:bool)
                n323 = Increment(x=w973) -> (x+1=w974:i32)
                n324 = Select(t=w974, s=w962, f=w973) -> (s? t:f=w972:i32)
              }
              frame 9 {
                w980 = TRUE  # PTO
                w987 = TRUE  # climbing
                w986 = FALSE  # pins in
                # "wait for robot to be secure on HAB"
                n325 = global read "Inputs_DriverStation.vi" "Master_Safety_Override"() -> (w988:bool)
                n326 = global read "SensorReadings.vi" "Robot On Ground"() -> (w976:bool)
                n327 = global read "Inputs_DriverStation.vi" "J1-Menu"() -> (w989:bool)
                n328 = Or(x=w976, y=w988) -> (x .or. y?=w984:bool)
                n329 = And(x=w989, y=w984) -> (x .and. y?=w979:bool)
                n330 = Increment(x=w982) -> (x+1=w983:i32)
                n331 = Select(t=w983, s=w979, f=w982) -> (s? t:f=w981:i32)
              }
              frame 10 {
                w995 = TRUE  # PTO
                w1001 = FALSE  # not climbing
                w1000 = FALSE  # pins in
                # "stop \"climbing\""
                n332 = Increment(x=w997) -> (x+1=w998:i32)
                n333 = Select(t=w998, s=TRUE, f=w997) -> (s? t:f=w996:i32)
              }
              frame 11 {
                w1005 = TRUE  # PTO
                w1013 = FALSE  # not climbing
                w1012 = FALSE  # pins in
                # "wait to disengage PTO"
                n334 = Increment(x=w1009) -> (x+1=w1010:i32)
                n335 = Select(t=w1010, s=TRUE, f=w1009) -> (s? t:f=w1008:i32)
              }
              frame 12 {
                w1031 = FALSE  # no PTO
                w1035 = FALSE  # not climbing
                w1034 = FALSE  # pins in
                # "retract legs"
                n336 = global read "Inputs_DriverStation.vi" "J1-Menu"() -> (w1015:bool)
                n337 = Not(x=w1015) -> (.not. x?=w1016:bool)
                n338 = feedback #17(FALSE ("PTO")) -> (w1019:bool)
                n339 = Select(t=TRUE ("no PTO"), s=w1016, f=w1019) -> (s? t:f=w1014:bool)
                n340 = feedback-in #17(w1014) -> ()
                n341 = And(x=w1014, y=w1015) -> (x .and. y?=w1017:bool)
                n342 = feedback #18(FALSE ("PTO")) -> (w1023:bool)
                n343 = Select(t=TRUE ("no PTO"), s=w1017, f=w1023) -> (s? t:f=w1021:bool)
                n344 = feedback-in #18(w1021) -> ()
                n345 = Increment(x=w1026) -> (x+1=w1027:i32)
                n346 = Select(t=w1027, s=w1021, f=w1026) -> (s? t:f=w1025:i32)
              }
              frame 13 {
                w1036 = TRUE  # end of match
                w1041 = FALSE  # no PTO
                w1045 = FALSE  # not climbing
                w1044 = FALSE  # pins in
                # "turn off the elevator"
              }
            }
          }
          frame 2 {
            w1049 = 57.0  # Level 3 PTO Okay
            w1051 = 62.0  # Level 3 Start
            w1063 = 60.0  # Level 3 PTO
            # "Level 3 buddy climb sequence"
            n347 = case shown="1" w1060 {
              selector: w1060 -> [w1074 w1090 w1106 w1124 w1136 w1158 w1172 w1185 w1205 w1214 w1227 w1239 w1257 w1270]
              tunnel: [w1076 w1092 w1101 w1123 w1135 w1157 w1171 w1184 w1204 w1213 w1226 w1238 w1256 w1270] -> w1054
              tunnel: [w1073 w1080 w1099 w1121 w1138 w1150 w1167 w1176 w1190 w1216 w1229 w1241 w1263 w1273] -> w1061
              tunnel: w1062 -> [_ w1080 w1099 _ w1138 w1150 w1167 _ w1190 w1216 w1229 w1241 w1263 w1273]
              tunnel: [w1072 w1089 w1112 w1122 w1134 w1160 w1174 w1187 w1207 w1217 w1230 w1242 w1264 w1274] -> w1055
              tunnel: [w1065 w1079 w1095 w1115 w1128 w1144 _ w1179 w1200 _ _ _ _ _] -> w1053
              tunnel: w1063 -> [_ _ _ _ _ _ w1164 w1179 w1200 _ _ _ _ _]
              tunnel: [w1070 w1088 w1100 w1119 w1133 w1153 w1170 w1183 w1203 w1218 w1231 w1243 w1265 w1275] -> w1056
              tunnel: [w1069 w1087 w1098 w1118 w1132 w1152 w1169 w1182 w1202 w1212 w1225 w1236 w1261 w1271] -> w1057
              tunnel: [FALSE FALSE FALSE FALSE FALSE FALSE FALSE FALSE FALSE FALSE TRUE TRUE TRUE FALSE] -> w1058
              tunnel: w1059 -> [_ _ _ _ _ _ _ _ _ _ _ _ _ _]
              tunnel: ["release mantis" "wait for mantis to deploy" "wait for elevator to reach climb height" "lock mantis" "confirm mantis lock" "wait for the driver to start climbing" "wait for elevator to pass PTO height" "engage the PTO" "ensure PTO is engaged" "wait for the robot to be on HAB" "stop climbing" "wait to disengage PTO" "retract the legs after confirm " "elevator powered down"] -> w1052
              tunnel: w1051 -> [_ _ w1095 w1115 w1128 w1144 _ _ _ _ _ _ _ _]
              tunnel: [-1.0 ("y") -1.0 ("y") -1.0 ("y") -1.0 ("y") -1.0 ("y") -1.0 ("y") -0.05 ("y") -0.05 ("y") -0.05 ("y") -1.0 ("y") -1.0 ("y") -1.0 ("y") -1.0 ("y") -1.0 ("y")] -> w1050
              tunnel: w1049 -> [_ _ _ _ _ _ _ _ w1196 _ _ _ _ _]
              tunnel: [_ _ _ _ _ _ _ _ _ _ _ _ _ w1267] -> w1048
              tunnel: w1047 -> [w1065 w1079 _ _ _ _ _ _ _ _ _ _ _ _]
              tunnel: [w1064 w1077 w1093 w1113 w1126 w1142 w1161 w1175 w1188 w1208 w1220 w1232 w1244 w1266] -> w1046
              frame 0, Default {
                w1064 = FALSE  # foot retracted
                w1069 = FALSE  # no PTO
                w1070 = FALSE  # not climbing
                w1072 = TRUE  # pins out
                # "release mantis pins and command to climb height"
                n348 = Increment(x=w1074) -> (x+1=w1075:i32)
                n349 = Select(t=w1075, s=TRUE, f=w1074) -> (s? t:f=w1076:i32)
                n350 = Tick Count (ms)() -> (millisecond timer value=w1073:u32)
              }
              frame 1 {
                w1077 = FALSE  # foot retracted
                w1087 = FALSE  # no PTO
                w1088 = FALSE  # not climbing
                w1089 = TRUE  # pins out
                # "wait for mantis to deploy"
                n351 = Tick Count (ms)() -> (millisecond timer value=w1083:u32)
                n352 = Subtract(x=w1083, y=w1080) -> (x-y=w1082:u32)
                n353 = Greater?(x=w1082, y=u32 250) -> (0:w1078:bool)
                n354 = Increment(x=w1090) -> (x+1=w1091:i32)
                n355 = Select(t=w1091, s=w1078, f=w1090) -> (s? t:f=w1092:i32)
              }
              frame 2 {
                w1093 = FALSE  # foot retracted
                w1098 = FALSE  # no PTO
                w1100 = FALSE  # not climbing
                w1112 = TRUE  # pins out
                # "wait for elevator to start moving\nand then stop moving"
                # "wait for elevator to reach climb position"
                n356 = global read "RobotStates.vi" "Elevator Moving"() -> (w1104:bool)
                n357 = call "RisingEdgeTrigger.vi"("Raw Signal"=w1104) -> ("Trigger"=w1111:bool)
                n358 = Not(x=w1104) -> (.not. x?=w1103:bool)
                n359 = feedback #19(FALSE) -> (w1109:bool)
                n360 = Select(t=TRUE, s=w1111, f=w1109) -> (s? t:f=w1105:bool)
                n361 = feedback-in #19(w1105) -> ()
                n362 = And(x=w1105, y=w1103) -> (x .and. y?=w1102:bool)
                n363 = Increment(x=w1106) -> (x+1=w1107:i32)
                n364 = Select(t=w1107, s=w1102, f=w1106) -> (s? t:f=w1101:i32)
              }
              frame 3 {
                w1113 = FALSE  # foot retracted
                w1118 = FALSE  # no PTO
                w1119 = FALSE  # not climbing
                w1122 = FALSE  # pins in
                # "lock mantis pins"
                n365 = Increment(x=w1124) -> (x+1=w1125:i32)
                n366 = Tick Count (ms)() -> (millisecond timer value=w1121:u32)
                n367 = Select(t=w1125, s=TRUE, f=w1124) -> (s? t:f=w1123:i32)
              }
              frame 4 {
                w1126 = FALSE  # foot retracted
                w1132 = FALSE  # no PTO
                w1133 = FALSE  # not climbing
                w1134 = FALSE  # pins in
                # "wait for mantis legs to lock"
                n368 = Tick Count (ms)() -> (millisecond timer value=w1141:u32)
                n369 = Subtract(x=w1141, y=w1138) -> (x-y=w1140:u32)
                n370 = Greater?(x=w1140, y=u32 500) -> (0:w1130:bool)
                n371 = Increment(x=w1136) -> (x+1=w1137:i32)
                n372 = Select(t=w1137, s=w1130, f=w1136) -> (s? t:f=w1135:i32)
              }
              frame 5 {
                w1142 = FALSE  # foot retracted
                w1152 = FALSE  # no PTO
                w1153 = FALSE  # not climbing
                w1160 = FALSE  # pins in
                # "wait for the driver to start climbing"
                n373 = global read "Inputs_DriverStation.vi" "J1-RightTrigger"() -> (w1149:dbl)
                n374 = Greater?(x=w1149, y=0.2) -> (0:w1147:bool)
                n375 = feedback #20(FALSE) -> (w1154:bool)
                n376 = Select(t=TRUE, s=w1147, f=w1154) -> (s? t:f=w1146:bool)
                n377 = feedback-in #20(w1146) -> ()
                n378 = Increment(x=w1158) -> (x+1=w1159:i32)
                n379 = Select(t=w1159, s=w1146, f=w1158) -> (s? t:f=w1157:i32)
              }
              frame 6 {
                w1161 = FALSE  # foot retracted
                w1169 = FALSE  # no PTO
                w1170 = TRUE  # climbing
                w1174 = FALSE  # pins in
                # "wait for elevator to pass PTO height"
                n380 = global read "SensorReadings.vi" "EncoderPos_Elevator"() -> (w1162:dbl)
                n381 = Less Or Equal?(x=w1162, y=w1164) -> (x <= y?=w1163:bool)
                n382 = Increment(x=w1172) -> (x+1=w1173:i32)
                n383 = Select(t=w1173, s=w1163, f=w1172) -> (s? t:f=w1171:i32)
              }
              frame 7 {
                w1175 = FALSE  # foot retracted
                w1182 = TRUE  # PTO
                w1183 = TRUE  # climbing
                w1187 = FALSE  # pins in
                # "engage the PTO"
                n384 = Increment(x=w1185) -> (x+1=w1186:i32)
                n385 = Tick Count (ms)() -> (millisecond timer value=w1176:u32)
                n386 = Select(t=w1186, s=TRUE, f=w1185) -> (s? t:f=w1184:i32)
              }
              frame 8 {
                w1188 = FALSE  # foot retracted
                w1202 = TRUE  # PTO
                w1203 = TRUE  # climbing
                w1207 = FALSE  # pins in
                # "timeout"
                # "ensure PTO is engaged"
                n387 = global read "SensorReadings.vi" "EncoderPos_Elevator"() -> (w1197:dbl)
                n388 = Tick Count (ms)() -> (millisecond timer value=w1193:u32)
                n389 = Less Or Equal?(x=w1197, y=w1196) -> (x <= y?=w1195:bool)
                n390 = Subtract(x=w1193, y=w1190) -> (x-y=w1192:u32)
                n391 = Greater?(x=w1192, y=u32 1000) -> (0:w1189:bool)
                n392 = Or(x=w1189, y=w1195) -> (x .or. y?=w1194:bool)
                n393 = Increment(x=w1205) -> (x+1=w1206:i32)
                n394 = Select(t=w1206, s=w1194, f=w1205) -> (s? t:f=w1204:i32)
              }
              frame 9 {
                w1208 = TRUE  # foot deployed
                w1212 = TRUE  # PTO
                w1218 = TRUE  # climbing
                w1217 = FALSE  # pins in
                # "wait for robot to be secure on HAB"
                n395 = global read "Inputs_DriverStation.vi" "J1-Menu"() -> (w1219:bool)
                n396 = Increment(x=w1214) -> (x+1=w1215:i32)
                n397 = Select(t=w1215, s=w1219, f=w1214) -> (s? t:f=w1213:i32)
              }
              frame 10 {
                w1220 = TRUE  # foot deployed
                w1225 = TRUE  # PTO
                w1231 = TRUE  # climbing
                w1230 = FALSE  # pins in
                # "******"
                # "stop \"climbing\""
                n398 = Increment(x=w1227) -> (x+1=w1228:i32)
                n399 = Select(t=w1228, s=TRUE, f=w1227) -> (s? t:f=w1226:i32)
              }
              frame 11 {
                w1232 = TRUE  # foot deployed
                w1236 = TRUE  # PTO
                w1243 = TRUE  # climbing
                w1242 = FALSE  # pins in
                # "******"
                # "wait to disengage PTO"
                n400 = Increment(x=w1239) -> (x+1=w1240:i32)
                n401 = Select(t=w1240, s=TRUE, f=w1239) -> (s? t:f=w1238:i32)
              }
              frame 12 {
                w1244 = TRUE  # foot deployed
                w1261 = FALSE  # no PTO
                w1265 = TRUE  # climbing
                w1264 = FALSE  # pins in
                # "*******"
                # "retract legs"
                n402 = global read "Inputs_DriverStation.vi" "J1-Menu"() -> (w1246:bool)
                n403 = Not(x=w1246) -> (.not. x?=w1247:bool)
                n404 = feedback #21(FALSE ("PTO")) -> (w1250:bool)
                n405 = Select(t=TRUE ("no PTO"), s=w1247, f=w1250) -> (s? t:f=w1245:bool)
                n406 = feedback-in #21(w1245) -> ()
                n407 = And(x=w1245, y=w1246) -> (x .and. y?=w1248:bool)
                n408 = feedback #22(FALSE ("PTO")) -> (w1254:bool)
                n409 = Select(t=TRUE ("no PTO"), s=w1248, f=w1254) -> (s? t:f=w1252:bool)
                n410 = feedback-in #22(w1252) -> ()
                n411 = Increment(x=w1257) -> (x+1=w1258:i32)
                n412 = Select(t=w1258, s=w1252, f=w1257) -> (s? t:f=w1256:i32)
              }
              frame 13 {
                w1266 = TRUE  # foot deployed
                w1267 = TRUE  # end of match
                w1271 = FALSE  # no PTO
                w1275 = TRUE  # climbing
                w1274 = FALSE  # pins in
                # "turn off the elevator"
              }
            }
          }
        }
      }
      n413 = feedback-in #8(w533) -> ()
      n414 = global write "RobotStates.vi" "Climb Sequence"(w528) -> ()
    }
  }
  "Target Elevator Position" <- w58
  "Target Vacuum Pump Power" <- w55
  n415 = feedback-in #5(w20) -> ()
  n416 = global write "RobotStates.vi" "Climb Sequence String"(w8) -> ()
  n417 = global write "SensorReadings.vi" "LimeLight In Range"(w5) -> ()
  n418 = global write "RobotStates.vi" "Climber Foot State"(w2) -> ()
  n419 = global write "SensorReadings.vi" "At HAB Height"(w9) -> ()
  n420 = global write "RobotStates.vi" "Max Climb Power"(w7) -> ()
  n421 = global write "RobotStates.vi" "End of Match"(w6) -> ()
  n422 = global write "RobotStates.vi" "PTO State"(w13) -> ()
  n423 = global write "RobotStates.vi" "Climb Started"(w14) -> ()
  n424 = global write "RobotStates.vi" "Climber Mantis State"(w1) -> ()
  n425 = global write "RobotStates.vi" "Upper Valve State"(w52) -> ()
  n426 = global write "RobotStates.vi" "Lower Valve State"(w51) -> ()
  n427 = global write "RobotStates.vi" "CARGO Intake Allowed"(w60) -> ()
  n428 = global write "RobotStates.vi" "CARGO Arm"(w59) -> ()
  n429 = global write "RobotStates.vi" "HATCH Arm"(w57) -> ()
  n430 = global write "RobotStates.vi" "HATCH Ejection Allowed"(w56) -> ()
  n431 = global read "Inputs_DriverStation.vi" "J1-View"() -> (w31:bool)
  n432 = Equal?(x=w29, y="Elevator_Stow") -> (x = y?=w45:bool)
  n433 = Equal?(x=w29, y="Cargo_Ground") -> (x = y?=w44:bool)
  n434 = Equal?(x=w29, y="Cargo_Feeder") -> (x = y?=w43:bool)
  n435 = Equal?(x=w29, y="Hatch_Ground") -> (x = y?=w42:bool)
  n436 = Equal?(x=w29, y="Hatch_Feeder") -> (x = y?=w41:bool)
  n437 = Equal?(x=w29, y="Climb") -> (x = y?=w40:bool)
  n438 = Compound Arithmetic op=OR(w45, w44, w43, w42, w41, w40, w31) -> (w37:bool)
  n439 = Not(x=w37) -> (.not. x?=w36:bool)
  n440 = while {
    shift-right: [w1280] -> w30
    shift-left: _ -> [w1281]
    tunnel: w36 -> [w1279]
    shift-right: [w1278] -> _
    shift-left: _ -> [w1277]
    tunnel: w29 -> [w1276]
    tunnel: [w1276] -> w28
    stop <- TRUE stop-if-true
    n441 = case shown="True" w1279 {
      tunnel: w1281 -> [_ w1288]
      tunnel: [0 w1287] -> w1280
      tunnel: [w1283 w1286] -> w1278
      tunnel: w1277 -> [w1283 w1285]
      frame False {
        # "stow, ground pickup, or feeder station"
      }
      frame True {
        # "rocket are cargo ship"
        n442 = case shown="1" w1288 {
          selector: w1288 -> [w1291 w1299 w1313 w1324 w1328 _]
          tunnel: [w1290 w1301 w1308 w1325 w1327 0 ("t")] -> w1287
          tunnel: [w1289 w1298 w1306 w1318 w1326 w1334] -> w1286
          tunnel: w1285 -> [w1289 _ w1306 _ w1326 w1334]
          frame 0, Default {
            # "wait for driver to start release"
            n443 = global read "Inputs_DriverStation.vi" "J1-LeftTrigger"() -> (w1294:dbl)
            n444 = Greater?(x=w1294, y=0.75) -> (0:w1292:bool)
            n445 = Increment(x=w1291) -> (x+1=w1295:i32)
            n446 = Select(t=w1295, s=w1292, f=w1291) -> (s? t:f=w1290:i32)
          }
          frame 1 {
            # "check for game piece release"
            n447 = global read "SensorReadings.vi" "Hatch Captured"() -> (w1304:bool)
            n448 = global read "SensorReadings.vi" "Cargo Captured"() -> (w1303:bool)
            n449 = Not(x=w1303) -> (.not. x?=w1297:bool)
            n450 = Not(x=w1304) -> (.not. x?=w1296:bool)
            n451 = Or(x=w1296, y=w1297) -> (x .or. y?=w1302:bool)
            n452 = Increment(x=w1299) -> (x+1=w1300:i32)
            n453 = Tick Count (ms)() -> (millisecond timer value=w1298:u32)
            n454 = Select(t=w1300, s=w1302, f=w1299) -> (s? t:f=w1301:i32)
          }
          frame 2 {
            # "***200"
            # "check to see if game piece actually gone"
            n455 = global read "SensorReadings.vi" "Hatch Captured"() -> (w1310:bool)
            n456 = global read "SensorReadings.vi" "Cargo Captured"() -> (w1311:bool)
            n457 = Tick Count (ms)() -> (millisecond timer value=w1317:u32)
            n458 = Subtract(x=w1317, y=w1306) -> (x-y=w1316:u32)
            n459 = Greater?(x=w1316, y=u32 0) -> (0:w1314:bool)
            n460 = Or(x=w1310, y=w1311) -> ()  [unwired: 1 out]
            n461 = Increment(x=w1313) -> (x+1=w1312:i32)
            n462 = Select(t=w1312, s=w1314, f=w1313) -> (s? t:f=w1309:i32)
            n463 = Select(t=0, s=FALSE, f=w1309) -> (s? t:f=w1308:i32)
          }
          frame 3 {
            # "wait for driver to release trigger"
            n464 = global read "Inputs_DriverStation.vi" "J1-LeftTrigger"() -> (w1322:dbl)
            n465 = Greater?(x=w1322, y=0.1) -> (0:w1320:bool)
            n466 = Not(x=w1320) -> (.not. x?=w1319:bool)
            n467 = Increment(x=w1324) -> (x+1=w1323:i32)
            n468 = Select(t=w1323, s=w1319, f=w1324) -> (s? t:f=w1325:i32)
            n469 = Tick Count (ms)() -> (millisecond timer value=w1318:u32)
          }
          frame 4 {
            # "safety wait"
            n470 = Tick Count (ms)() -> (millisecond timer value=w1333:u32)
            n471 = Subtract(x=w1333, y=w1326) -> (x-y=w1332:u32)
            n472 = Greater?(x=w1332, y=u32 50) -> (0:w1330:bool)
            n473 = Increment(x=w1328) -> (x+1=w1329:i32)
            n474 = Select(t=w1329, s=w1330, f=w1328) -> (s? t:f=w1327:i32)
          }
          frame 5 {
            # "trigger auto stow"
            n475 = global write "RobotStates.vi" "Auto Stow"(TRUE) -> ()
          }
        }
      }
    }
  }
  "Elevator State Out" <- w28
  n476 = global write "RobotStates.vi" "Auto Stow Sequence"(w30) -> ()
